vi "Simple H5Awrite_GenerateCode.vi"(1 "Terms":T13[](array[typedef]), 3 "Diagram":refnum<vi>, 5 "XRef":refnum<vi>, 6 "State In":T1) -> (0 "Generated Code?":bool, 2 "State Out":T1, 4 "Reply":string[](array[string]))   [LabVIEW 2017, in "Simple H5Awrite.xnode"]
uses:
  <vilib>/UPVI/lvhdf5/attribute.llb/Simple H5Awrite.xnode
  <vilib>/XNodeSupport/XNodeTermIDPair.ctl
  <vilib>/XNodeSupport/XNodeTermRef.ctl
  <vilib>/XNodeSupport/XNodeString.ctl
  <vilib>/UPVI/lvhdf5/attribute.llb/Simple H5Awrite/Simple H5Awrite_State.ctl
  <vilib>/UPVI/lvhdf5/xnodehelpers/TermsPlus.ctl
  <vilib>/XNodeSupport/XNodeTerm3.ctl
  <vilib>/XNodeSupport/XNodeVariant.ctl
  <vilib>/XNodeSupport/XNodeRect32.ctl
  <vilib>/XNodeSupport/XNodeInt.ctl
  <vilib>/XNodeSupport/XNodeBool.ctl
  <vilib>/XNodeSupport/XNodeTermDirection.ctl
  <vilib>/UPVI/lvhdf5/xnodehelpers/TermBehavior.ctl
  <vilib>/XNodeSupport/XNodeError3Array.ctl
  <vilib>/XNodeSupport/XNodeError3.ctl
  <vilib>/XNodeSupport/NI_XNodeSupport.lvlib
panel:
  in  "vi path":path
  # "LVHDF5 Toolkit\nCopyright (c) 2005-2013 by Jason D. Sommerville\nCopyright (c) 2014 by UPVI, LLC.\n\nThis use and distribution of this file is governed by the terms found in \nLICENSE.txt distributed with this toolkit and installed at\n <user.lib>\\_lvhdf5\\LICENSE.txt"
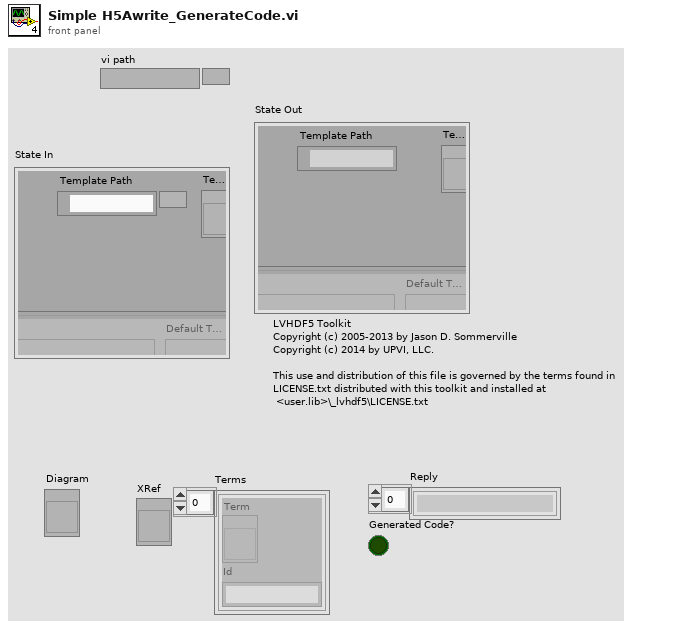
[diagram p1: front panel]
types:
  T1 = typedef "Simple H5Awrite.xnode/Simple H5Awrite_State.ctl" = cluster{"Template Path":path, "Template Ref":refnum<vi>, "Terms":T2[], "Display Name":string, "Image":picture, "Errors":T11, "Generated?":bool}
  T2 = typedef "TermsPlus.ctl" = cluster{"Term 3":T3, "Default Type":variant, "Behavior":T10, "Behavior Arg":string, "WiredResponse":bool, "Wired":enum16{"Unknown", "Unwired", "Wired"}}
  T3 = typedef "NI_XNodeSupport.lvlib/XNodeTerm3.ctl" = cluster{"Name":T4, "Id":T4, "Type":T5, "Bounds":T6, "Input?":T8, "Required?":T8, "Recommended?":T8, "Adaptive?":T8, "Hidden?":T8, "Direction":T9, "Break Wire?":T8}
  T4 = typedef "NI_XNodeSupport.lvlib/XNodeString.ctl" = string
  T5 = typedef "NI_XNodeSupport.lvlib/XNodeVariant.ctl" = variant
  T6 = typedef "NI_XNodeSupport.lvlib/XNodeRect32.ctl" = cluster{"Left":T7, "Top":T7, "Right":T7, "Bottom":T7}
  T7 = typedef "NI_XNodeSupport.lvlib/XNodeInt.ctl" = i32
  T8 = typedef "NI_XNodeSupport.lvlib/XNodeBool.ctl" = bool
  T9 = typedef "NI_XNodeSupport.lvlib/XNodeTermDirection.ctl" = enum32{"Auto", "Up", "Down", "Left", "Right", "Center"}
  T10 = typedef "TermBehavior.ctl" = enum16{"Normal", "Anything", "LVType", "Path or Ref", "Attr Name", "Attr Poly", "Elt Poly", "Dset Poly", "WDT Poly"}
  T11 = typedef "NI_XNodeSupport.lvlib/XNodeError3Array.ctl" = T12[]
  T12 = typedef "NI_XNodeSupport.lvlib/XNodeError3.ctl" = cluster{"Error":T4, "Details":T4, "Help File":T4, "Help Topic":T4}
  T13 = typedef "NI_XNodeSupport.lvlib/XNodeTermIDPair.ctl" = cluster{"Term":T14, "Id":T4}
  T14 = typedef "NI_XNodeSupport.lvlib/XNodeTermRef.ctl" = refnum<vi>
  T15 = typedef "LVPositionTypeDef.ctl" = cluster{"Left":i32, "Top":i32}
  T16 = typedef "NI_XNodeSupport.lvlib/XNodeStringArray.ctl" = T4[]
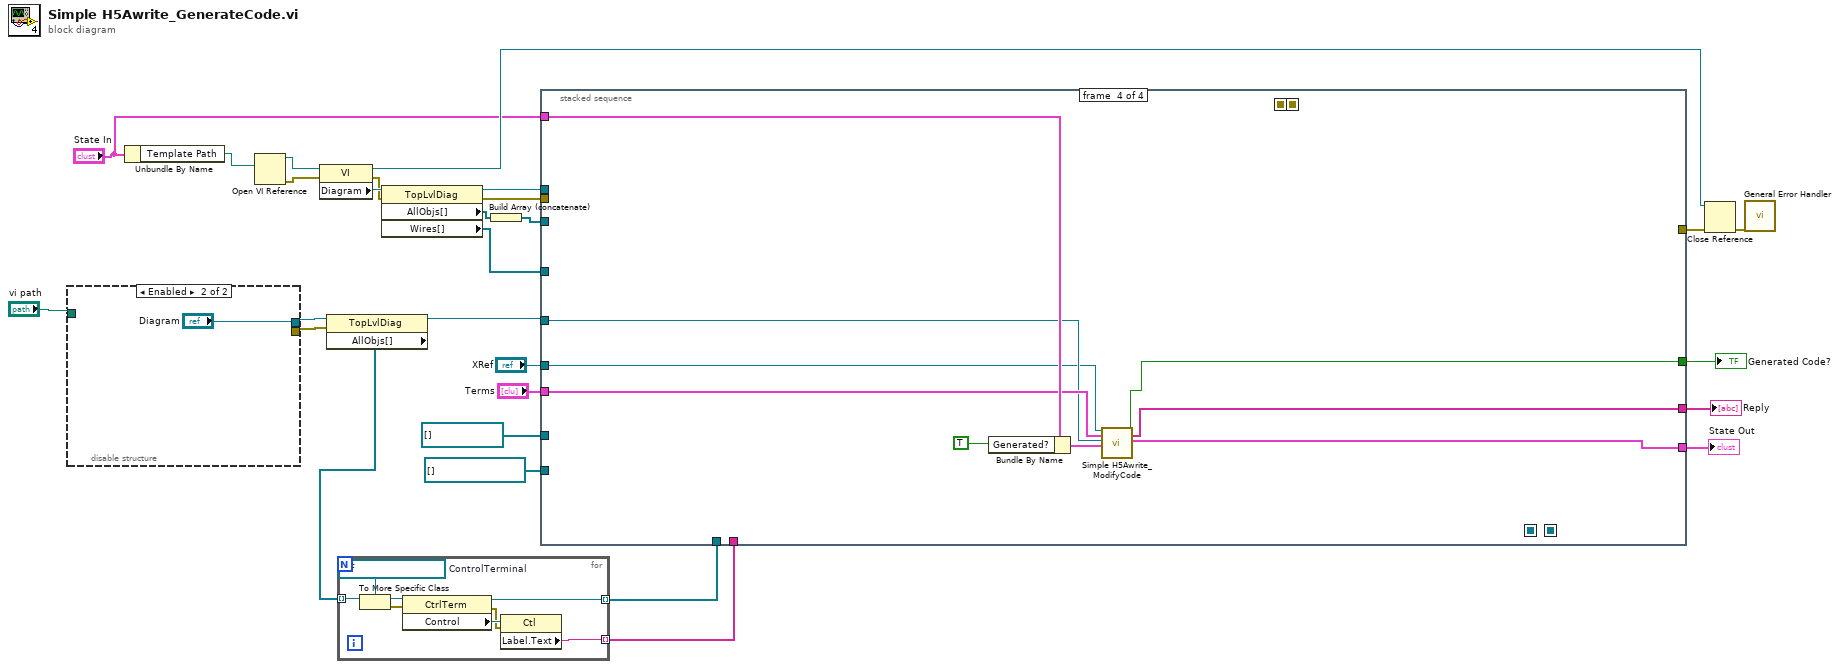
[diagram p0: block diagram]
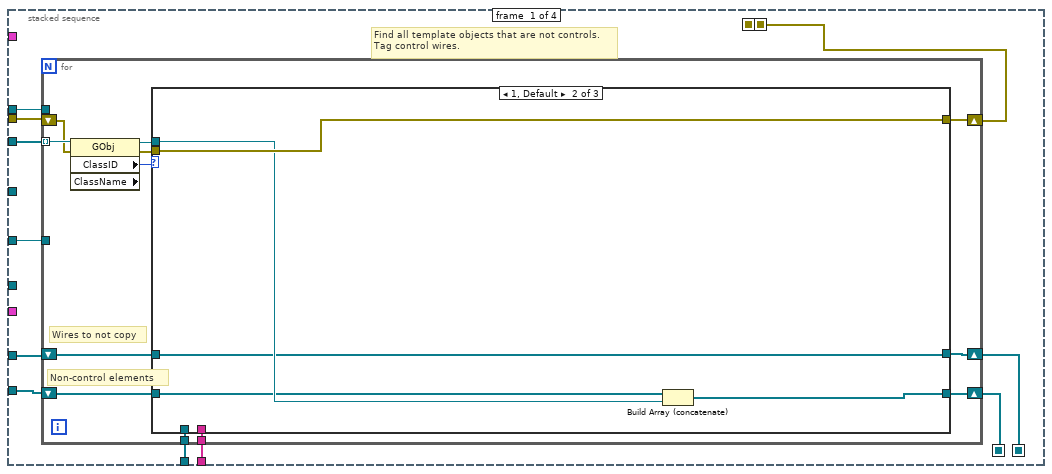
[diagram p2: hidden frame]
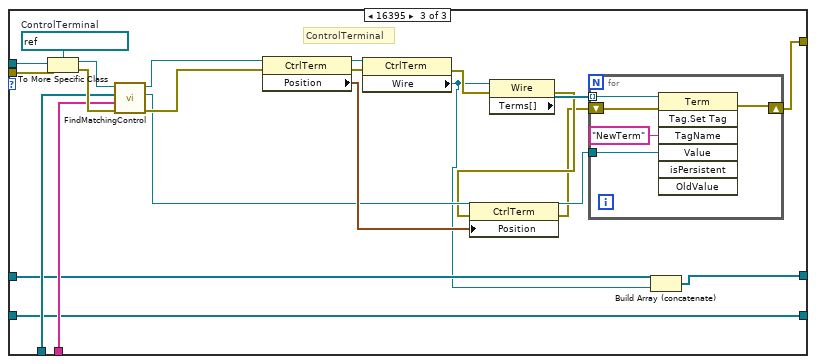
[diagram p4: hidden frame]
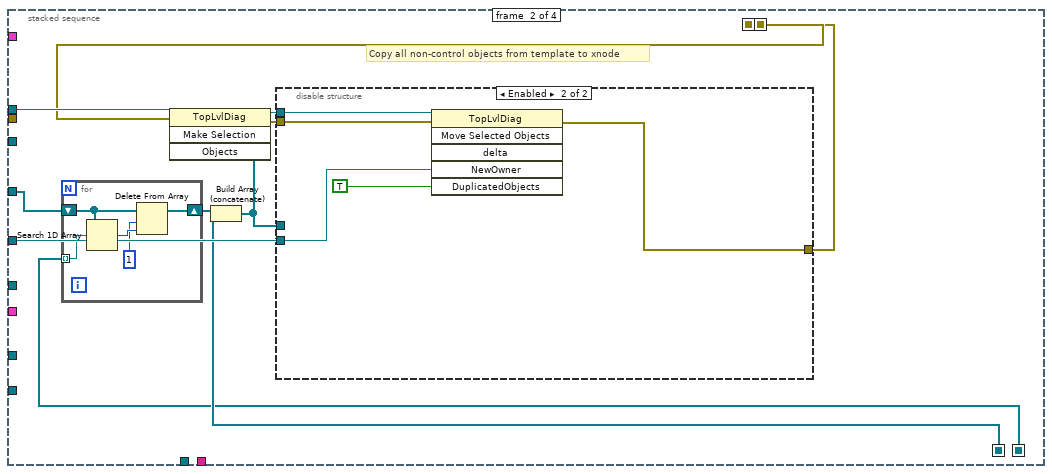
[diagram p5: hidden frame]
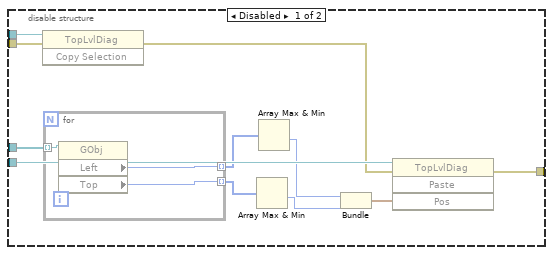
[diagram p6: hidden frame]
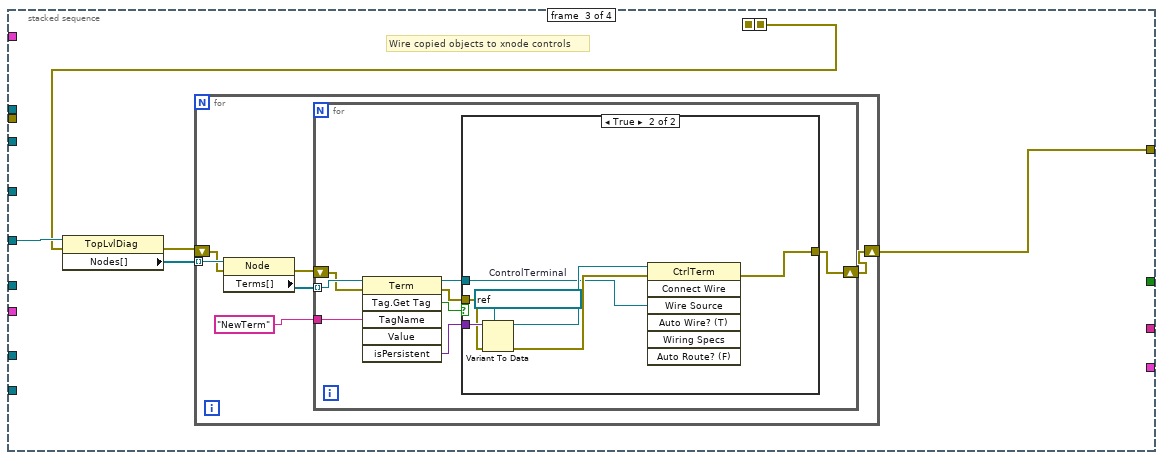
[diagram p7: hidden frame]
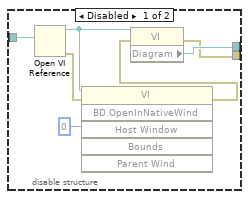
[diagram p9: hidden frame]
diagram:
  n1 = disable-structure shown="Enabled" {
    disable-tunnel: "vi path" -> [w35 _]
    disable-tunnel: [w34 "Diagram"] -> w24
    disable-tunnel: [w33 _] -> w15
    frame Disabled {
      n2 = Open VI Reference(vi path=w35) -> (vi reference=w32:refnum<vi>, error out=w31:errorcluster)  [unwired: 5 in]
      n3 = invoke class="VI" method="BD.OpenInNativeWind"(reference=w32, error in=w31, "Host Window"=u64 0) -> (error out=w30:errorcluster)  [unwired: 3 in, 5 out]
      n4 = property class="VI"(reference=w32, error in=w30) -> (error out=w33:errorcluster, "Diagram"=w34:refnum<vi>)  [unwired: 1 out]
    }
    frame Enabled {
    }
  }
  n5 = Unbundle By Name("State In") -> ("Template Path"=w14:path)
  n6 = Open VI Reference(vi path=w14) -> (vi reference=w12:refnum<vi>, error out=w13:errorcluster)  [unwired: 5 in]
  n7 = property class="VI"(reference=w12, error in=w13) -> (reference out=w9:refnum<vi>, error out=w25:errorcluster, "Diagram"=w28:refnum<vi>)
  n8 = property class="TopLvlDiag"(reference=w24, error in=w15) -> (reference out=w17:refnum<vi>, "AllObjs[]"=w23:refnum<vi>[])  [unwired: 1 out]
  n9 = for {
    tunnel: w23 -> [w44] mode=indexing
    tunnel: [w39] -> w18 mode=indexing
    tunnel: [w38] -> w19 mode=indexing
    w43 = refnum<vi> refnum  # ControlTerminal
    n10 = To More Specific Class(target class=w43, reference=w44) -> (specific class reference=w42:refnum<vi>, error out=w37:errorcluster)  [unwired: 1 in]
    n11 = property class="CtrlTerm"(reference=w42, error in=w37) -> (reference out=w38:refnum<vi>, error out=w40:errorcluster, "Control"=w41:refnum<vi>)
    n12 = property class="Ctl"(reference=w41, error in=w40) -> ("Label.Text"=w39:string)  [unwired: 2 out]
  }
  n13 = property class="TopLvlDiag"(reference=w28, error in=w25) -> (reference out=w22:refnum<vi>, error out=w21:errorcluster, "AllObjs[]"=w26:refnum<vi>[], "Wires[]"=w8:refnum<vi>[])
  n14 = Build Array (concatenate)(w26) -> (w20:refnum<vi>[])
  n15 = stacked-sequence {
    seq-local: [w48 _ _ _] -> [_ w106 _ _]
    seq-local: [w51 _ _ _] -> [_ w110 _ _]
    seq-local: [_ w109 _ _] -> [_ _ w140 _]
    seq-local: [w45 _ _ _] -> [_ w104 _ _]
    tunnel: w20 -> [w55 _ _ _]
    tunnel: w22 -> [w54 w114 _ _]
    tunnel: w21 -> [w49 _ _ _]
    tunnel: w18 -> [w53 _ _ _]
    tunnel: w17 -> [w52 w111 w141 w170]
    tunnel: w19 -> [w50 _ _ _]
    tunnel: [_ _ w139 _] -> w11
    tunnel: refnum<vi>[] [] -> [w47 _ _ _]
    tunnel: w8 -> [_ w108 _ _]
    tunnel: refnum<vi>[] [] -> [w46 _ _ _]
    tunnel: "State In" -> [_ _ _ w173]
    tunnel: "Terms" -> [_ _ _ w171]
    tunnel: "XRef" -> [_ _ _ w169]
    tunnel: [_ _ _ w168] -> w3
    tunnel: [_ _ _ w167] -> w2
    tunnel: [_ _ _ w166] -> w1
    frame #0 {
      # "Find all template objects that are not controls.\nTag control wires."
      n16 = for {
        tunnel: w55 -> [w67] mode=indexing
        tunnel: w54 -> [_]
        shift-right: [w60] -> w51
        shift-left: w49 -> [w66]
        tunnel: w53 -> [w61]
        tunnel: w52 -> [_]
        tunnel: w50 -> [w62]
        shift-right: [w59] -> w48
        shift-left: w47 -> [w58]
        shift-right: [w56] -> w45
        shift-left: w46 -> [w57]
        # "Wires to not copy"
        # "Non-control elements"
        n17 = property class="GObj" props=["ClassID", "ClassName"](reference=w67, error in=w66) -> (reference out=w63:refnum<vi>, error out=w64:errorcluster, "ClassID"=w65:u32)  [unwired: 1 out]
        n18 = case shown="1, Default" w65 {
          tunnel: w63 -> [_ w74 w97]
          tunnel: w64 -> [w70 w75 w96]
          tunnel: w61 -> [_ _ w86]
          tunnel: [w70 w75 w79] -> w60
          tunnel: w62 -> [_ _ w87]
          tunnel: [w69 w73 w85] -> w59
          tunnel: w58 -> [w69 w72 w85]
          tunnel: w57 -> [w68 w71 w78]
          tunnel: [w68 w71 w76] -> w56
          frame 0 {
          }
          frame 1, Default {
            n19 = Build Array (concatenate)(w72, w74) -> (w73:refnum<vi>[])
          }
          frame 16395 {
            w98 = refnum<vi> refnum  # ControlTerminal
            # "ControlTerminal"
            n20 = To More Specific Class(target class=w98, reference=w97, error in=w96) -> (specific class reference=w94:refnum<vi>, error out=w95:errorcluster)
            n21 = call <vilib>:"FindMatchingControl.vi"("error in"=w95, "ControlNames"=w86, "ControlIDs"=w87, "Source Ctrl Ref"=w94) -> ("error out"=w91:errorcluster, "Target Ctrl Ref"=w88:refnum<vi>, "Source Ctrl Ref out"=w93:refnum<vi>)  [unwired: 1 in, 2 out]
            n22 = property class="CtrlTerm"(reference=w93, error in=w91) -> (reference out=w90:refnum<vi>, error out=w89:errorcluster, "Position"=w92:T15)
            n23 = property class="CtrlTerm"(reference=w90, error in=w89) -> (error out=w83:errorcluster, "Wire"=w77:refnum<vi>)  [unwired: 1 out]
            n24 = property class="Wire"(reference=w77, error in=w83) -> (error out=w82:errorcluster, "Terms[]"=w84:refnum<vi>[])  [unwired: 1 out]
            n25 = property class="CtrlTerm"(reference=w88, error in=w82, "Position"=w92) -> (reference out=w81:refnum<vi>, error out=w80:errorcluster)
            n26 = for {
              tunnel: w84 -> [w103] mode=indexing
              shift-right: [w101] -> w79
              shift-left: w80 -> [w102]
              tunnel: w81 -> [w100]
              n27 = invoke class="Term" method="Tag.Set Tag"(reference=w103, error in=w102, "TagName"="NewTerm" ("Tag Name"), "Value"=w100) -> (error out=w101:errorcluster)  [unwired: 3 in, 6 out]
            }
            n28 = Build Array (concatenate)(w78, w77) -> (w76:refnum<vi>[])
          }
        }
      }
    }
    frame #1 {
      # "Copy all non-control objects from template to xnode"
      n29 = for {
        shift-right: [w115] -> w107
        shift-left: w108 -> [w116]
        tunnel: w104 -> [w119] mode=indexing
        n30 = Search 1D Array(1D array=w116, element=w119) -> (index of element=w118:i32)  [unwired: 1 in]
        n31 = Delete From Array(array=w116, length=1, index=w118) -> (array with subset deleted=w115:refnum<vi>[])  [unwired: 1 out]
      }
      n32 = Build Array (concatenate)(w107, w106) -> (w105:refnum<vi>[])
      n33 = invoke class="TopLvlDiag" method="Make Selection"(reference=w114, error in=w110, "Objects"=w105) -> (reference out=w113:refnum<vi>, error out=w112:errorcluster)  [unwired: 1 in, 2 out]
      n34 = disable-structure shown="Enabled" {
        disable-tunnel: w113 -> [w130 w138]
        disable-tunnel: w112 -> [w129 w137]
        disable-tunnel: w111 -> [w128 w136]
        disable-tunnel: [w126 w134] -> w109
        disable-tunnel: w105 -> [w120 _]
        frame Disabled {
          n35 = invoke class="TopLvlDiag" method="Copy Selection"(reference=w130, error in=w129) -> (error out=w127:errorcluster)  [unwired: 1 in, 2 out]
          n36 = for {
            tunnel: w120 -> [w133] mode=indexing
            tunnel: [w132] -> w124 mode=indexing
            tunnel: [w131] -> w125 mode=indexing
            n37 = property class="GObj"(reference=w133) -> ("Left"=w132:i32, "Top"=w131:i32)  [unwired: 1 in, 2 out]
          }
          n38 = Array Max & Min(array=w125) -> (min value=w122:i32)  [unwired: 3 out]
          n39 = Array Max & Min(array=w124) -> (min value=w123:i32)  [unwired: 3 out]
          n40 = Bundle(w123, w122) -> (w121:cluster{i32, i32})  [unwired: 1 in]
          n41 = invoke class="TopLvlDiag" method="Paste"(reference=w128, error in=w127, "Pos"=w121) -> (error out=w126:errorcluster)  [unwired: 1 in, 3 out]
        }
        frame Enabled {
          n42 = invoke class="TopLvlDiag" method="Move Selected Objects"(reference=w138, error in=w137, "NewOwner"=w136, "DuplicatedObjects"=TRUE ("Duplicate?")) -> (error out=w134:errorcluster)  [unwired: 2 in, 5 out]
        }
      }
    }
    frame #2 {
      # "Wire copied objects to xnode controls"
      n43 = property class="TopLvlDiag"(reference=w141, error in=w140) -> (error out=w142:errorcluster, "Nodes[]"=w143:refnum<vi>[])  [unwired: 1 out]
      n44 = for {
        tunnel: w143 -> [w149] mode=indexing
        shift-right: [w145] -> w139
        shift-left: w142 -> [w146]
        n45 = property class="Node"(reference=w149, error in=w146) -> (error out=w144:errorcluster, "Terms[]"=w148:refnum<vi>[])  [unwired: 1 out]
        n46 = for {
          tunnel: w148 -> [w154] mode=indexing
          tunnel: "NewTerm" ("Tag Name") -> [w157]
          shift-right: [w152] -> w145
          shift-left: w144 -> [w151]
          n47 = invoke class="Term" method="Tag.Get Tag"(reference=w154, error in=w151, "TagName"=w157) -> (reference out=w150:refnum<vi>, error out=w155:errorcluster, "GetTag"=w153:bool, "isPersistent"=w156:variant)  [unwired: 3 in, 2 out]
          n48 = case shown="True" w153 {
            tunnel: [w158 w162] -> w152
            tunnel: w156 -> [_ w161]
            tunnel: w155 -> [w158 w160]
            tunnel: w150 -> [_ w159]
            frame False {
            }
            frame True {
              w165 = refnum<vi> refnum  # ControlTerminal
              n49 = Variant To Data(error in=w160, type=w165, Variant=w161) -> (data=w164:refnum<vi>, error out=w163:errorcluster)
              n50 = invoke class="CtrlTerm" method="Connect Wire"(reference=w164, error in=w163, "Wire Source"=w159) -> (error out=w162:errorcluster)  [unwired: 4 in, 6 out]
            }
          }
        }
      }
    }
    frame #3 {
      n51 = Bundle By Name(cluster=w173, "Generated?"=TRUE ("Generated Code?")) -> (w172:T1)
      n52 = call <vilib>:"Simple H5Awrite_ModifyCode.vi"("XRef"=w169, "Terms"=w171, "Diagram"=w170, "State In"=w172) -> ("Generated Code?"=w166:T8, "Reply"=w167:T16, "State Out"=w168:T1)  [unwired: 13 in]
    }
  }
  "Reply" <- w2
  "Generated Code?" <- w1
  "State Out" <- w3
  n53 = Close Reference(reference=w9, error in (no error)=w11) -> (error out=w10:errorcluster)
  n54 = call <vilib>:"General Error Handler.vi"("error in (no error)"=w10) -> ()  [unwired: 10 in, 5 out]
